vi "LSM9DS1_Open.vi"(6 "NumCalSamples":i32, 8 "error in (no error)":errorcluster, 9 "Accel-Gyro_Settings":T4={"Accel_Range"=enum."±4g", "Gyro_Range"=enum."±500dps", "A/G_Address"=enum."0x6B", "Motion Thresh"=0.0, "reset"=FALSE}, 10 "Mag_Settings":T5={"Mag_Range"=enum."±2 gauss", "Mag_Address"=enum."0x1E", "Anomaly Thresh"=0.0, "Local Mag"=0.0}, 11 "I2C Bus":T3=enum."Invalid") -> (0 "error out":errorcluster, 1 "IMU Cal Result":T1, 3 "LSM9DS1DevRef Out":T2={"DevStatus"={"status"=FALSE, "code"=0, "source"=""}, "Gyro Offset"={"Xzero"=0.0, "Yzero"=0.0, "Zzero"=0.0}, "StdDev Rates"={"Xsdo"=0.0, "Ysdo"=0.0, "Zsdo"=0.0}, "Reset"=FALSE, "Accel Offset"={"Xzero"=0.0, "Yzero"=0.0, "Zzero"=0.0}, "Motion Thresh"=0.0, "Mag Offset"={"Xzero"=0.0, "Yzero"=0.0, "Zzero"=0.0}, "I2C Bus"=enum."I2C On-Board", "Handle"=0, "Anomaly Thresh"=0.0, "Local Mag"=0.0, "Accel/Gyro_Address"=enum."0x6B", "Accel_Range"=enum."±4g", "Gyro_Range"=enum."±500dps", "Mag_Range"=enum."±2 gauss", "Mag_Address"=enum."0x1E", "accel_active"=FALSE, "gyro_active"=FALSE, "mag_active"=FALSE})   [LabVIEW 2015]
uses:
  <vilib>/Rock Robotics/SystemInterfaces/i2clib/i2c_bus.ctl
  LSM9DS1DevRef.ctl
  <vilib>/Analysis/NI_AALBase.lvlib
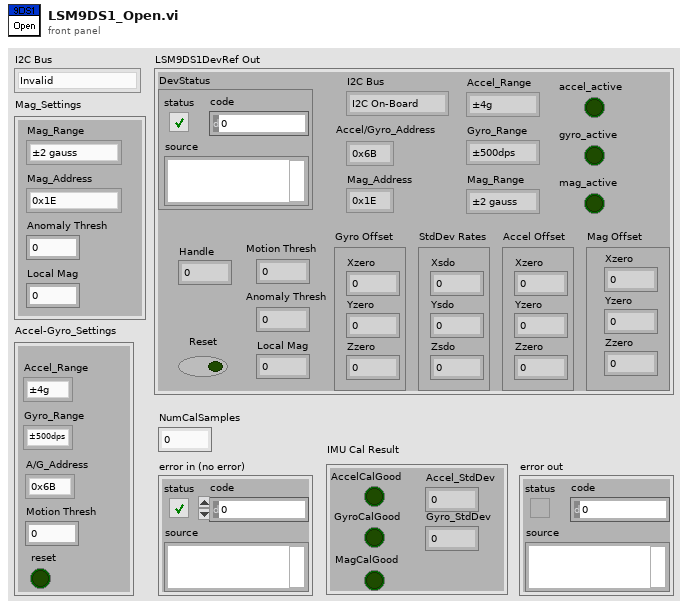
[diagram p1: front panel]
types:
  T1 = cluster{"AccelCalGood":bool, "GyroCalGood":bool, "MagCalGood":bool, "Accel_StdDev":dbl, "Gyro_StdDev":dbl}
  T2 = typedef "LSM9DS1DevRef.ctl" = cluster{"DevStatus":errorcluster, "Gyro Offset":cluster{"Xzero":dbl, "Yzero":dbl, "Zzero":dbl}, "StdDev Rates":cluster{"Xsdo":dbl, "Ysdo":dbl, "Zsdo":dbl}, "Reset":bool, "Accel Offset":cluster{"Xzero":dbl, "Yzero":dbl, "Zzero":dbl}, "Motion Thresh":dbl, "Mag Offset":cluster{"Xzero":dbl, "Yzero":dbl, "Zzero":dbl}, "I2C Bus":T3, "Handle":i32, "Anomaly Thresh":dbl, "Local Mag":dbl, "Accel/Gyro_Address":enum8{"0x6A", "0x6B"}, "Accel_Range":enum16{"±2g", "±16g", "±4g", "±8g", "disabled"}, "Gyro_Range":enum16{"±245dps", "±500dps", "disabled", "±2000dps"}, "Mag_Range":enum16{"±2 gauss", "±4 gauss", "±8 gauss", "±16 gauss", "disabled"}, "Mag_Address":enum8{"0x1C", "0x1E"}, "accel_active":bool, "gyro_active":bool, "mag_active":bool}
  T3 = typedef "i2c_bus.ctl" = enum16{"I2C On-Board", "I2C MXP", "Invalid"}
  T4 = cluster{"Accel_Range":enum8{"±2g", "±16g", "±4g", "±8g", "disabled"}, "Gyro_Range":enum8{"±245dps", "±500dps", "disabled", "±2000dps"}, "A/G_Address":enum8{"0x6A", "0x6B"}, "Motion Thresh":dbl, "reset":bool}
  T5 = cluster{"Mag_Range":enum8{"±2 gauss", "±4 gauss", "±8 gauss", "±16 gauss", "disabled"}, "Mag_Address":enum8{"0x1C", "0x1E"}, "Anomaly Thresh":dbl, "Local Mag":dbl}
  T6 = typedef "WPI_I2CDevRef.ctl" = cluster{"DevStatus":errorcluster, "Device Address":u8, "Handle":i32, "I2C Bus":T3}
  T7 = enum8{"±2 gauss", "±4 gauss", "±8 gauss", "±16 gauss", "disabled"}
  T8 = enum8{"±245dps", "±500dps", "disabled", "±2000dps"}
  T9 = cluster{"AccelCalGood":bool, "GyroCalGood":bool, "MagCalGood":bool, "Gyro_StdDev":dbl, "Accel_StdDev":dbl}
  T10 = typedef "Gyro_TypeDef.ctl" = cluster{"Pitch":dbl, "Yaw":dbl, "X Ang Rate":dbl, "Y Ang Rate":dbl, "Z Ang Rate":dbl, "Roll":dbl}
  T11 = typedef "Accel_TypeDef.ctl" = cluster{"X Accel":dbl, "Y Accel":dbl, "Z Accel":dbl, "Pitch":dbl, "Roll":dbl}
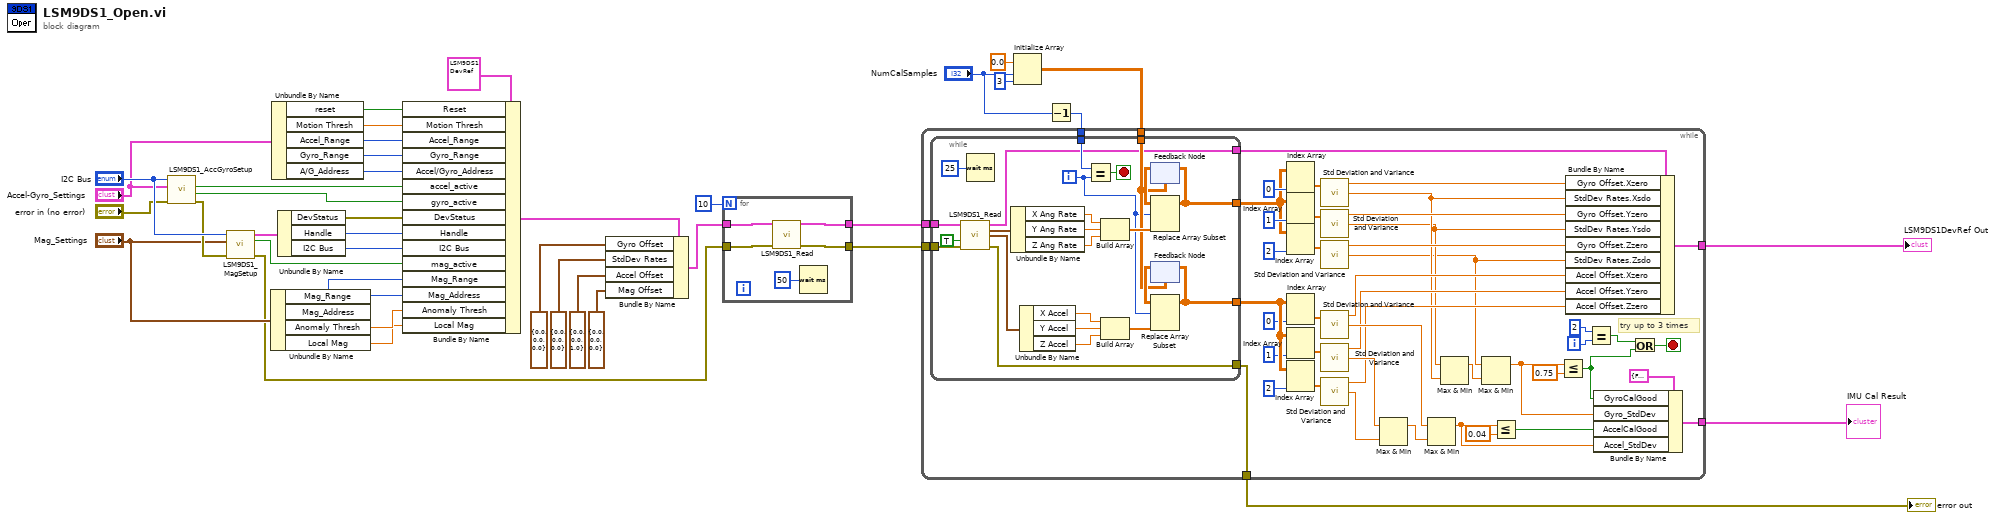
[diagram p0: block diagram]
diagram:
  n1 = call "LSM9DS1_AccGyroSetup.vi"("error in (no error)"="error in (no error)", "Accel-Gyro_Settings"="Accel-Gyro_Settings", "I2C Bus"="I2C Bus") -> ("error out"=w38:errorcluster, "Gyro_Active"=w33:bool, "Accel_Active"=w34:bool)  [unwired: 5 in, 1 out]
  n2 = call "LSM9DS1_MagSetup.vi"("error in (no error)"=w38, "Mag_Settings"="Mag_Settings", "I2C Bus"="I2C Bus") -> ("error out"=w12:errorcluster, "Mag_Active"=w29:bool, "I2CMagDevRef"=w37:T6)  [unwired: 6 in]
  n3 = Unbundle By Name("Mag_Settings") -> ("Mag_Range"=w26:T7, "Mag_Address"=w25:enum8{"0x1C", "0x1E"}, "Anomaly Thresh"=w22:dbl, "Local Mag"=w21:dbl)
  n4 = Unbundle By Name("Accel-Gyro_Settings") -> ("reset"=w19:bool, "Motion Thresh"=w20:dbl, "Accel_Range"=w28:enum8{"±2g", "±16g", "±4g", "±8g", "disabled"}, "Gyro_Range"=w27:T8, "A/G_Address"=w36:enum8{"0x6A", "0x6B"})
  n5 = Unbundle By Name(w37) -> ("DevStatus"=w32:errorcluster, "Handle"=w31:i32, "I2C Bus"=w30:T3)
  n6 = Bundle By Name(cluster=T2 {"DevStatus"={"status"=FALSE, "code"=0, "source"=""}, "Gyro Offset"={"Xzero"=0.0, "Yzero"=0.0, "Zzero"=0.0}, "StdDev Rates"={"Xsdo"=0.0, "Ysdo"=0.0, "Zsdo"=0.0}, "Reset"=FALSE, "Accel Offset"={"Xzero"=0.0, "Yzero"=0.0, "Zzero"=0.0}, "Motion Thresh"=0.0, "Mag Offset"={"Xzero"=0.0, "Yzero"=0.0, "Zzero"=0.0}, "I2C Bus"=enum."I2C On-Board", "Handle"=0, "Anomaly Thresh"=0.0, "Local Mag"=0.0, "Accel/Gyro_Address"=enum."0x6B", "Accel_Range"=enum."±4g", "Gyro_Range"=enum."±500dps", "Mag_Range"=enum."±2 gauss", "Mag_Address"=enum."0x1E", "accel_active"=FALSE, "gyro_active"=FALSE, "mag_active"=FALSE} ("LSM9DS1DevRef"), "Reset"=w19, "Motion Thresh"=w20, "Accel_Range"=w28, "Gyro_Range"=w27, "Accel/Gyro_Address"=w36, "accel_active"=w34, "gyro_active"=w33, "DevStatus"=w32, "Handle"=w31, "I2C Bus"=w30, "mag_active"=w29, "Mag_Range"=w26, "Mag_Address"=w25, "Anomaly Thresh"=w22, "Local Mag"=w21) -> (w18:T2)
  n7 = Bundle By Name(cluster=w18, "Gyro Offset"=cluster{"Xzero":dbl, "Yzero":dbl, "Zzero":dbl} {"Xzero"=0.0, "Yzero"=0.0, "Zzero"=0.0}, "StdDev Rates"=cluster{"Xsdo":dbl, "Ysdo":dbl, "Zsdo":dbl} {"Xsdo"=0.0, "Ysdo"=0.0, "Zsdo"=0.0}, "Accel Offset"=cluster{"Xzero":dbl, "Yzero":dbl, "Zzero":dbl} {"Xzero"=0.0, "Yzero"=0.0, "Zzero"=1.0}, "Mag Offset"=cluster{"Xzero":dbl, "Yzero":dbl, "Zzero":dbl} {"Xzero"=0.0, "Yzero"=0.0, "Zzero"=0.0}) -> (w11:T2)
  n8 = for {
    N: 10 -> [_]
    tunnel: w12 -> [w44]
    tunnel: [w43] -> w9
    tunnel: w11 -> [w42]
    tunnel: [w41] -> w10
    n9 = call "LSM9DS1_Read.vi"("LSM9DS1DevRef"=w42, "error in (no error)"=w44) -> ("LSM9DS1DevRef Out"=w41:T2, "error out"=w43:errorcluster)  [unwired: 8 in, 4 out]
    n10 = Wait (ms)(milliseconds to wait=u32 50) -> ()  [unwired: 1 out]
  }
  n11 = Initialize Array(0.0 ("element"), "NumCalSamples", 3 ("dimension size")) -> (w6:dbl[][])
  n12 = Decrement(x="NumCalSamples") -> (x-1=w4:i32)
  n13 = while {
    tunnel: w10 -> [w92]
    tunnel: w9 -> [w91]
    tunnel: w6 -> [w90]
    tunnel: w4 -> [w89]
    tunnel: [w61] -> w3
    tunnel: [w56] -> w2
    tunnel: [w55] -> w1
    i -> [w54]
    stop <- w52 stop-if-true
    # "try up to 3 times"
    n14 = while {
      tunnel: w92 -> [w116]
      tunnel: w91 -> [w115]
      tunnel: w90 -> [w102]
      tunnel: w89 -> [w100]
      tunnel: [w98] -> w55
      tunnel: [w97] -> w72
      tunnel: [w95] -> w85
      tunnel: [w94] -> w73
      i -> [w99]
      stop <- w101 stop-if-true
      n15 = call "LSM9DS1_Read.vi"("LSM9DS1DevRef"=w116, "Reset"=TRUE, "error in (no error)"=w115) -> ("LSM9DS1DevRef Out"=w97:T2, "Gyro"=w114:T10, "Accel"=w103:T11, "error out"=w98:errorcluster)  [unwired: 7 in, 2 out]
      n16 = Wait (ms)(milliseconds to wait=u32 25) -> ()  [unwired: 1 out]
      n17 = Unbundle By Name(w114) -> ("X Ang Rate"=w113:dbl, "Y Ang Rate"=w112:dbl, "Z Ang Rate"=w111:dbl)
      n18 = Unbundle By Name(w103) -> ("X Accel"=w108:dbl, "Y Accel"=w107:dbl, "Z Accel"=w106:dbl)
      n19 = Equal?(x=w100, y=w99) -> (x = y?=w101:bool)
      n20 = Build Array(w113, w112, w111) -> (w110:dbl[])
      n21 = Build Array(w108, w107, w106) -> (w105:dbl[])
      n22 = feedback #1(w102) -> (w109:dbl[][])
      n23 = Replace Array Subset(array=w109, new element=w110, index (row)=w99) -> (w94:dbl[][])  [unwired: 1 in]
      n24 = feedback-in #1(w94) -> ()
      n25 = feedback #2(w102) -> (w104:dbl[][])
      n26 = Replace Array Subset(array=w104, new element=w105, index (row)=w99) -> (w95:dbl[][])  [unwired: 1 in]
      n27 = feedback-in #2(w95) -> ()
    }
    n28 = Index Array(array=w73, index (col)=0 ("disabled index (col)")) -> (element=w80:dbl[])  [unwired: 1 in]
    n29 = Index Array(array=w73, index (col)=1 ("disabled index (col)")) -> (element=w79:dbl[])  [unwired: 1 in]
    n30 = Index Array(array=w73, index (col)=2 ("disabled index (col)")) -> (element=w78:dbl[])  [unwired: 1 in]
    n31 = Index Array(array=w85, index (col)=0 ("disabled index (col)")) -> (element=w88:dbl[])  [unwired: 1 in]
    n32 = Index Array(array=w85, index (col)=1 ("disabled index (col)")) -> (element=w87:dbl[])  [unwired: 1 in]
    n33 = Index Array(array=w85, index (col)=2 ("disabled index (col)")) -> (element=w86:dbl[])  [unwired: 1 in]
    n34 = call <vilib>:"Std Deviation and Variance.vi"("X"=w80) -> ("mean"=w67:dbl, "standard deviation"=w60:dbl)  [unwired: 1 in, 1 out]
    n35 = call <vilib>:"Std Deviation and Variance.vi"("X"=w79) -> ("mean"=w66:dbl, "standard deviation"=w59:dbl)  [unwired: 1 in, 1 out]
    n36 = call <vilib>:"Std Deviation and Variance.vi"("X"=w78) -> ("mean"=w65:dbl, "standard deviation"=w57:dbl)  [unwired: 1 in, 1 out]
    n37 = call <vilib>:"Std Deviation and Variance.vi"("X"=w88) -> ("mean"=w64:dbl, "standard deviation"=w69:dbl)  [unwired: 1 in, 1 out]
    n38 = call <vilib>:"Std Deviation and Variance.vi"("X"=w87) -> ("mean"=w63:dbl, "standard deviation"=w70:dbl)  [unwired: 1 in, 1 out]
    n39 = call <vilib>:"Std Deviation and Variance.vi"("X"=w86) -> ("mean"=w62:dbl, "standard deviation"=w71:dbl)  [unwired: 1 in, 1 out]
    n40 = Max & Min(x=w70, y=w71) -> (max(x,y)=w68:dbl)  [unwired: 1 out]
    n41 = Max & Min(x=w69, y=w68) -> (max(x,y)=w46:dbl)  [unwired: 1 out]
    n42 = Max & Min(x=w59, y=w60) -> (max(x,y)=w58:dbl)  [unwired: 1 out]
    n43 = Max & Min(x=w57, y=w58) -> (max(x,y)=w48:dbl)  [unwired: 1 out]
    n44 = Less Or Equal?(x=w46, y=0.04) -> (x <= y?=w47:bool)
    n45 = Less Or Equal?(x=w48, y=0.75) -> (x <= y?=w50:bool)
    n46 = Bundle By Name(cluster=w72, "Gyro Offset.Xzero"=w67, "StdDev Rates.Xsdo"=w60, "Gyro Offset.Yzero"=w66, "StdDev Rates.Ysdo"=w59, "Gyro Offset.Zzero"=w65, "StdDev Rates.Zsdo"=w57, "Accel Offset.Xzero"=w64, "Accel Offset.Yzero"=w63, "Accel Offset.Zzero"=w62) -> (w56:T2)
    n47 = Equal?(x=2, y=w54) -> (x = y?=w51:bool)
    n48 = Bundle By Name(cluster=T9 {"AccelCalGood"=FALSE, "GyroCalGood"=FALSE, "MagCalGood"=FALSE, "Gyro_StdDev"=0.0, "Accel_StdDev"=0.0} ("input cluster"), "GyroCalGood"=w50, "Gyro_StdDev"=w48, "AccelCalGood"=w47, "Accel_StdDev"=w46) -> (w61:T9)
    n49 = Or(x=w51, y=w50) -> (x .or. y?=w52:bool)
  }
  "error out" <- w1
  "LSM9DS1DevRef Out" <- w2
  "IMU Cal Result" <- w3
